vi "Periodic Tasks.vi"(8 "error in (no error)":errorcluster) -> ()   [LabVIEW 2013]
doc: "This VI runs in parallel to other tasks. It can contain as many user-defined periodic loops as you need. These can carry out PID or other sorts of timed response."
uses:
  <vilib>/Rock Robotics/SystemInterfaces/AI/FPGA_AIGyroChannel.ctl
  <vilib>/Rock Robotics/SystemInterfaces/Typedef/FPGA_TypedefAnalogModuleForGyro.ctl
  PnuematicMode.ctl
  TankDriveEnum.ctl
  <vilib>/Rock Robotics/SystemInterfaces/Utilities/FPGA_UtilitiesLED Source.ctl
  <vilib>/Rock Robotics/SystemInterfaces/Utilities/FPGA_UtilitiesLED State.ctl
  Robot Global Data.vi
  <vilib>/Rock Robotics/WPI/Compressor/WPI_CompressorGetSetRefNum.vi
panel:
  out "Angular Rate":dbl
  in  "Analog Module":T1
  in  "Gain (VoltsPerDegree/Second)":dbl=0.007
  in  "Channel":T2
  in  "Reset Zero Position":bool
  out "Angle":dbl(knob) scale=0.0..360.0
  out "error out":errorcluster
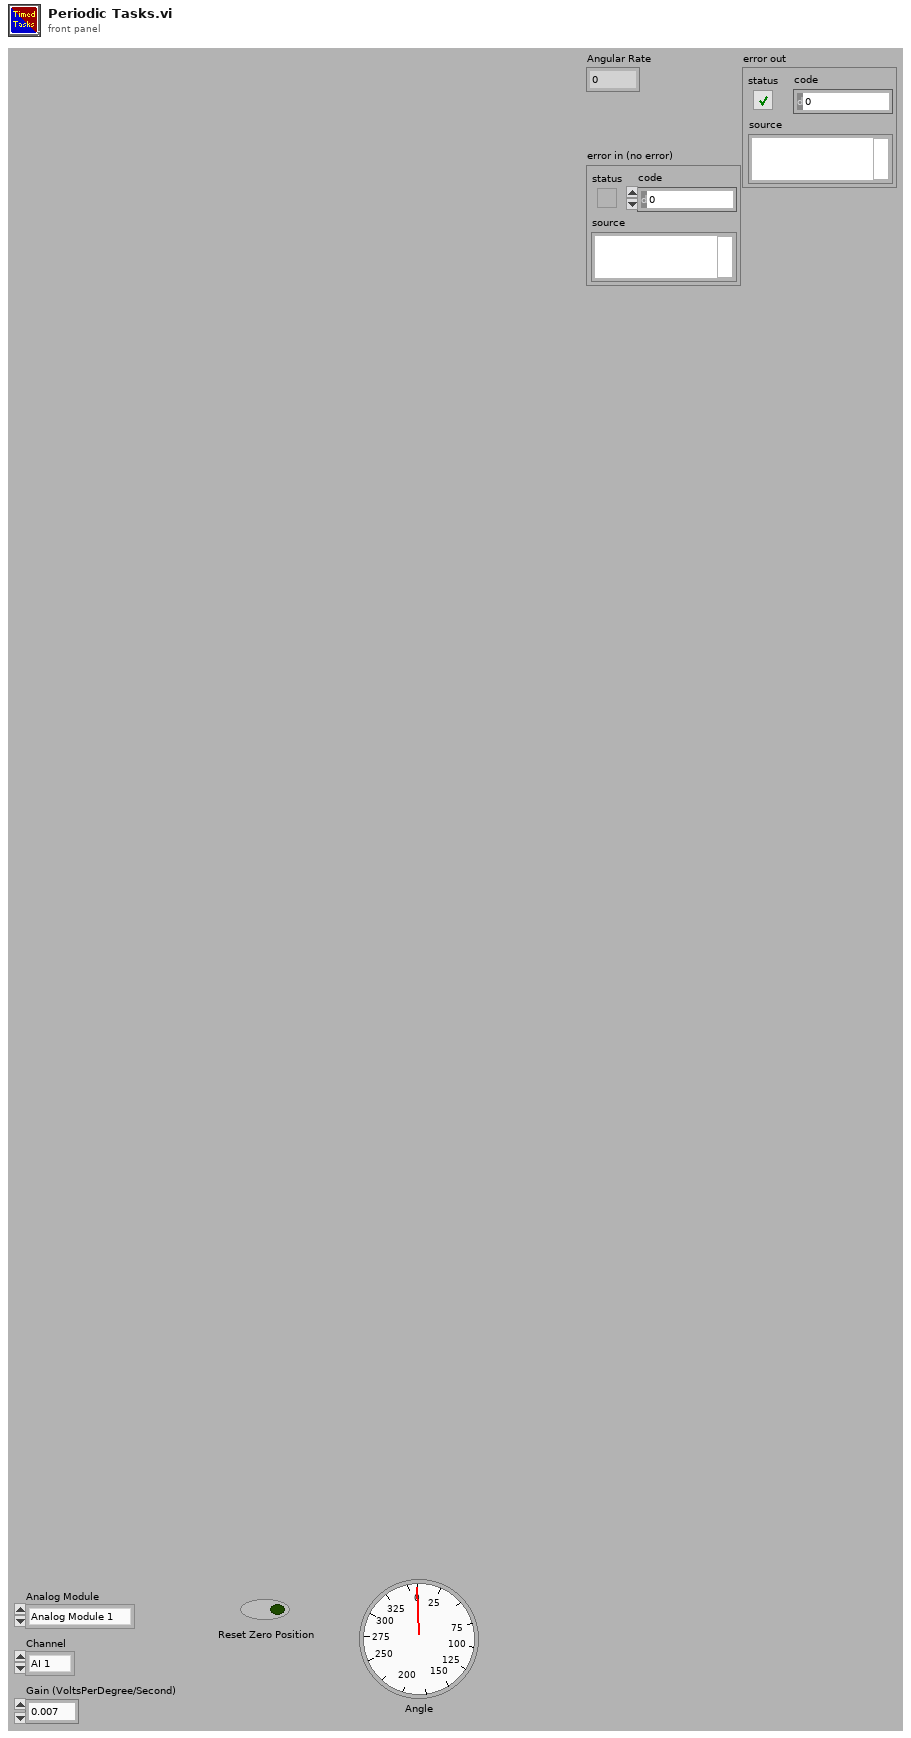
[diagram p1: front panel]
types:
  T1 = typedef "FPGA_TypedefAnalogModuleForGyro.ctl" = enum16{"Analog Module 1"}
  T2 = typedef "FPGA_AIGyroChannel.ctl" = enum8{"AI 1", "AI 2", "Invalid"}
  T3 = typedef "WPI_EncoderDevRef.ctl" = cluster{"DevStatus":errorcluster, "EncoderIndex":T4, "CounterIndex":T5, "DistancePerCount":dbl, "Decoding Type":T6}
  T4 = typedef "FPGA_EncoderIdx.ctl" = enum8{"Enc 0", "Enc 1", "Enc 2", "Enc 3", "Invalid"}
  T5 = typedef "FPGA_CounterCtrSystemIndex.ctl" = enum8{"Ctr 0", "Ctr 1", "Ctr 2", "Ctr 3", "Ctr 4", "Ctr 5", "Ctr 6", "Ctr 7", "Invalid"}
  T6 = typedef "WPI_EncoderType.ctl" = enum16{"1x", "2x", "4x"}
  T7 = typedef "WPI_GyroDevRef.ctl" = cluster{"DevStatus":errorcluster, "Analog Module":T8, "Analog Channel":T9, "Offset":dbl, "Gain (VoltsPerDegree/Second)":dbl}
  T8 = typedef "FPGA_TypedefAnalogModule.ctl" = enum16{"Analog Module 1", "Analog Module 2"}
  T9 = typedef "FPGA_AIChannel.ctl" = enum8{"AI 1", "AI 2", "AI 3", "AI 4", "AI 5", "AI 6", "AI 7", "AI 8", "Invalid"}
  T10 = typedef "WPI_SolenoidDevRef.ctl" = cluster{"DevStatus":errorcluster, "Solenoid Module":T11, "Forward Solenoid Channel":T12, "Reverse Solenoid Channel":T12}
  T11 = typedef "FPGA_TypedefSolenoidModule.ctl" = enum16{"Solenoid Module 1", "Solenoid Module 2"}
  T12 = typedef "WPI_SolenoidChannel.ctl" = enum8{"Solenoid 1", "Solenoid 2", "Solenoid 3", "Solenoid 4", "Solenoid 5", "Solenoid 6", "Solenoid 7", "Solenoid 8", "Invalid"}
  T13 = typedef "WPI_CompressorDevRef.ctl" = cluster{"DevStatus":errorcluster, "DigitalInputDevRef":T14, "RelayDevRef":T17}
  T14 = typedef "WPI_DigitalInputDevRef.ctl" = cluster{"DevStatus":errorcluster, "DIO Channel":T15, "Digital Module":T16}
  T15 = typedef "FPGA_DIOChannel.ctl" = enum8{"DIO 1", "DIO 2", "DIO 3", "DIO 4", "DIO 5", "DIO 6", "DIO 7", "DIO 8", "DIO 9", "DIO 10", "DIO 11", "DIO 12", "DIO 13", "DIO 14", "Invalid"}
  T16 = typedef "FPGA_TypedefDigitalModule.ctl" = enum16{"Digital Module 1", "Digital Module 2"}
  T17 = typedef "WPI_RelayDevRef.ctl" = cluster{"DevStatus":errorcluster, "Relay Channel":T18, "Digital Module":T16, "Relay Direction":T19}
  T18 = typedef "FPGA_DIORelayChannel.ctl" = enum8{"Relay 1", "Relay 2", "Relay 3", "Relay 4", "Relay 5", "Relay 6", "Relay 7", "Relay 8", "Invalid"}
  T19 = typedef "WPI_RelayDirection.ctl" = enum16{"Both directions", "Forward only", "Reverse only"}
  T20 = typedef "TankDriveEnum.ctl" = enum16{"Init", "LinearDrive", "SetValue", "Disable"}
  T21 = typedef "PnuematicMode.ctl" = enum16{"Init", "SetState", "Disable"}
  T22 = typedef "FPGA_UtilitiesLED State.ctl" = enum16{"Off", "On", "Toggle"}
  T23 = typedef "FPGA_UtilitiesLED Source.ctl" = enum16{"User LED", "FPGA LED"}
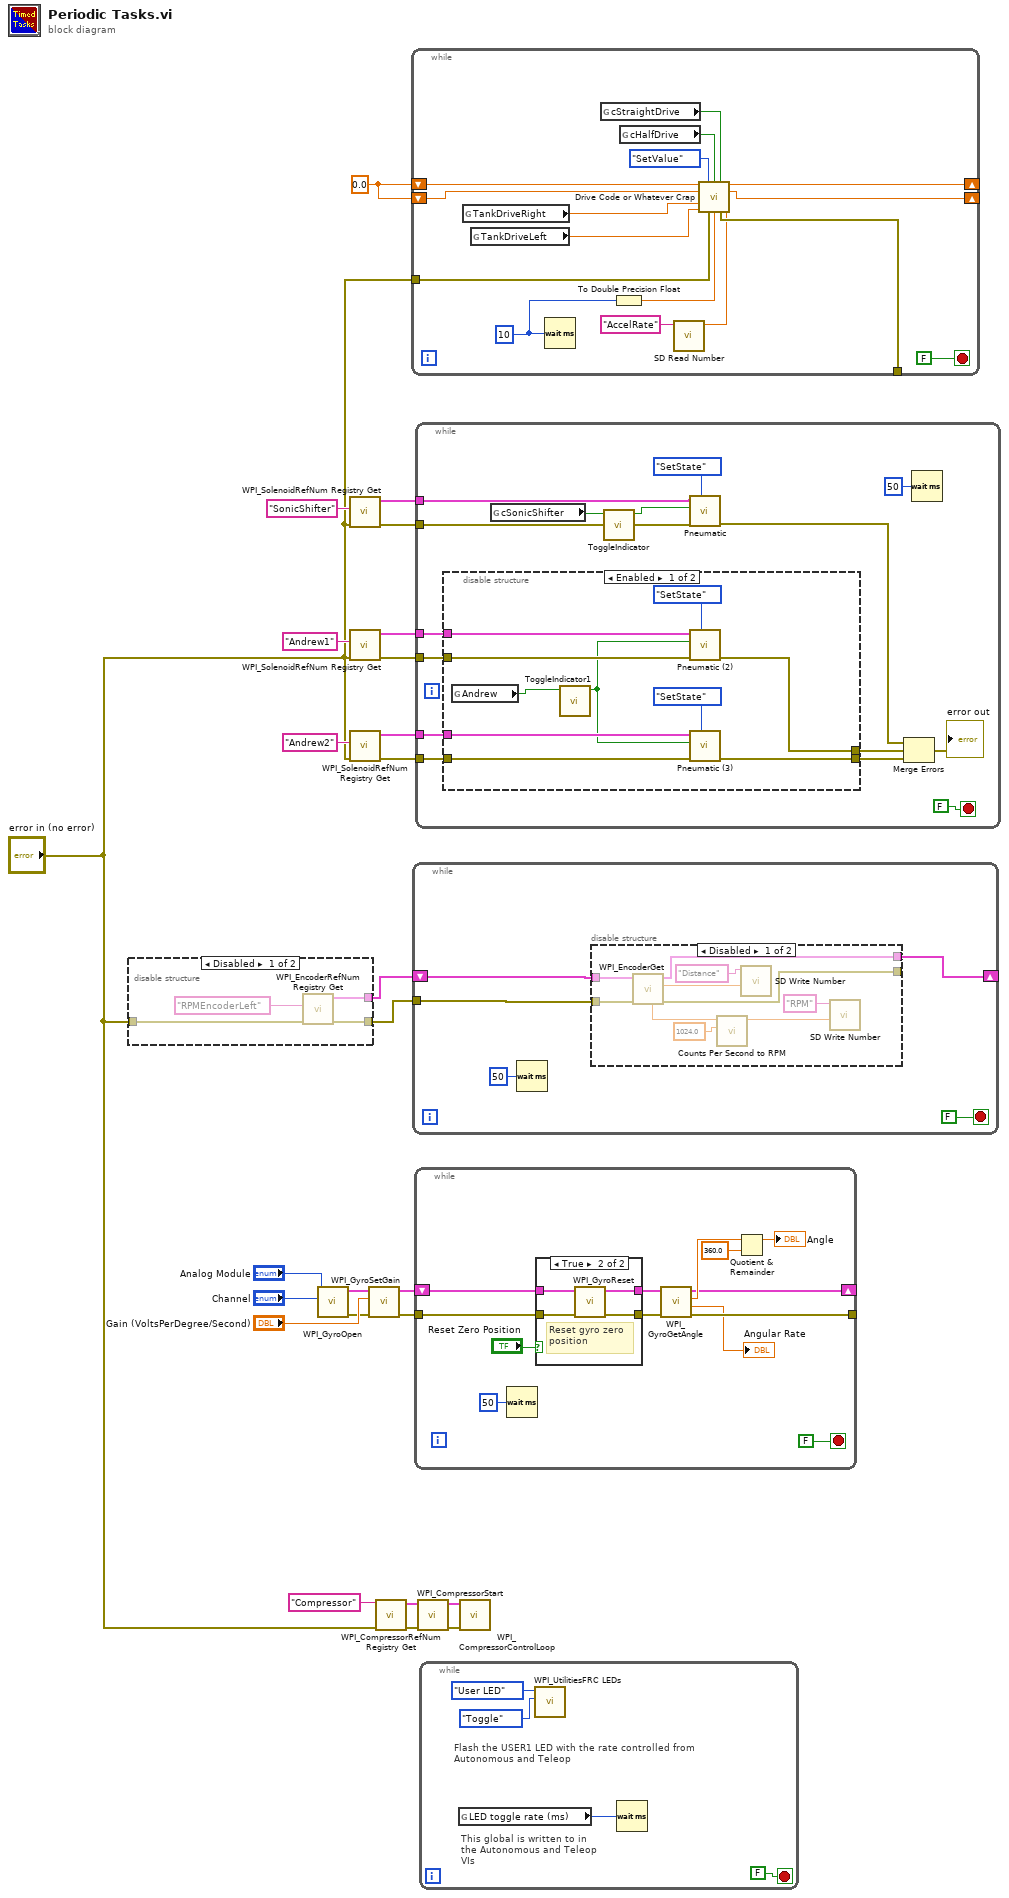
[diagram p0: block diagram]
diagram:
  w11 = 0.0
  n1 = disable-structure shown="Disabled" {
    disable-tunnel: [w28 _] -> w9
    disable-tunnel: [w27 _] -> w8
    disable-tunnel: "error in (no error)" -> [w26 _]
    frame Disabled {
      n2 = call <vilib>:"WPI_EncoderRefNum Registry Get.vi"("error in (no error)"=w26, "refnum name"="RPMEncoderLeft") -> ("error out"=w27:errorcluster, "EncoderDevRef"=w28:T3)  [unwired: 8 in]
    }
    frame Enabled {
    }
  }
  n3 = call <vilib>:"WPI_GyroOpen.vi"("Analog Channel"="Channel", "Analog Module (Module 1)"="Analog Module") -> ("error out"=w2:errorcluster, "GyroDevRef"=w6:T7)  [unwired: 4 in, 4 out]
  n4 = call <vilib>:"WPI_SolenoidRefNum Registry Get.vi"("error in (no error)"="error in (no error)", "refnum name"="SonicShifter") -> ("error out"=w18:errorcluster, "SolenoidDevRef"=w20:T10)  [unwired: 8 in]
  n5 = call <vilib>:"WPI_SolenoidRefNum Registry Get.vi"("error in (no error)"="error in (no error)", "refnum name"="Andrew1") -> ("error out"=w13:errorcluster, "SolenoidDevRef"=w15:T10)  [unwired: 8 in]
  n6 = call <vilib>:"WPI_SolenoidRefNum Registry Get.vi"("error in (no error)"="error in (no error)", "refnum name"="Andrew2") -> ("error out"=w12:errorcluster, "SolenoidDevRef"=w14:T10)  [unwired: 8 in]
  n7 = call <vilib>:"WPI_GyroSetGain.vi"("error in (no error)"=w2, "Gain (VoltsPerDegree/Second)"="Gain (VoltsPerDegree/Second)", "GyroDevRef"=w6) -> ("error out"=w1:errorcluster, "GyroDevRef"=w5:T7)  [unwired: 7 out]
  n8 = call <vilib>:"WPI_CompressorRefNum Registry Get.vi"("error in (no error)"="error in (no error)", "refnum name"="Compressor") -> ("error out"=w22:errorcluster, "CompressorDevRef"=w25:T13)  [unwired: 8 in]
  n9 = while {
    shift-right: [w39] -> _
    shift-left: w11 -> [w40]
    shift-right: [w38] -> _
    shift-left: w11 -> [w41]
    tunnel: "error in (no error)" -> [w37]
    tunnel: [w36] -> _
    stop <- FALSE stop-if-true
    w35 = u32 10 ("milliseconds to wait")
    n10 = global read "Robot Global Data.vi" "TankDriveRight"() -> (w45:dbl)
    n11 = global read "Robot Global Data.vi" "TankDriveLeft"() -> (w44:dbl)
    n12 = Wait (ms)(milliseconds to wait=w35) -> ()  [unwired: 1 out]
    n13 = global read "Robot Global Data.vi" "cStraightDrive"() -> (w42:bool)
    n14 = To Double Precision Float(number=w35) -> (double precision float=w34:dbl)
    n15 = global read "Robot Global Data.vi" "cHalfDrive"() -> (w43:bool)
    n16 = call <vilib>:"SD Read Number.vi"("Name"="AccelRate") -> ("Numeric"=w31:dbl)  [unwired: 8 in, 2 out]
    n17 = call "Drive Code or Whatever Crap.vi"("Right Actual"=w40, "TankDriveEnum"=TankDriveEnum."SetValue" ("Enum"), "HalfDrive"=w43, "StraightDrive"=w42, "LeftActual"=w41, "RightDesired"=w45, "LeftDesired"=w44, "error in (no error)"=w37, "LoopTime"=w34, "AccelRate"=w31) -> ("RightOut"=w39:dbl, "LeftOut"=w38:dbl, "error out"=w36:errorcluster)  [unwired: 3 in]
  }
  n18 = while {
    tunnel: w8 -> [w47]
    shift-right: [w46] -> _
    shift-left: w9 -> [w48]
    stop <- FALSE stop-if-true
    n19 = Wait (ms)(milliseconds to wait=u32 50) -> ()  [unwired: 1 out]
    n20 = disable-structure shown="Disabled" {
      disable-tunnel: w47 -> [w60 _]
      disable-tunnel: w48 -> [w53 _]
      disable-tunnel: [w52 _] -> _
      disable-tunnel: [w51 _] -> w46
      frame Disabled {
        n21 = call <vilib>:"WPI_EncoderGet.vi"("error in (no error)"=w60, "EncoderDevRef"=w53) -> ("error out"=w52:errorcluster, "Distance"=w55:dbl, "EncoderDevRef"=w51:T3, "Rate"=w59:dbl)  [unwired: 4 in, 2 out]
        n22 = call "Counts Per Second to RPM.vi"("Counts/Rev"=1024.0, "Counts/Second"=w59) -> ("RPM"=w57:dbl)  [unwired: 9 in]
        n23 = call <vilib>:"SD Write Number.vi"("Numeric"=w55, "Name"="Distance") -> ()  [unwired: 8 in, 2 out]
        n24 = call <vilib>:"SD Write Number.vi"("Numeric"=w57, "Name"="RPM") -> ()  [unwired: 8 in, 2 out]
      }
      frame Enabled {
      }
    }
  }
  n25 = while {
    shift-right: [w69] -> _
    shift-left: w5 -> [w72]
    tunnel: w1 -> [w65]
    tunnel: [w63] -> _
    stop <- FALSE stop-if-true
    n26 = Wait (ms)(milliseconds to wait=u32 50) -> ()  [unwired: 1 out]
    n27 = case shown="True" "Reset Zero Position" {
      tunnel: w72 -> [w74 w78]
      tunnel: [w74 w77] -> w71
      tunnel: w65 -> [_ w76]
      tunnel: [_ w75] -> w64
      frame False {
      }
      frame True {
        # "Reset gyro zero \nposition"
        n28 = call <vilib>:"WPI_GyroReset.vi"("error in (no error)"=w76, "GyroDevRef"=w78) -> ("error out"=w75:errorcluster, "GyroDevRef"=w77:T7)  [unwired: 8 out]
      }
    }
    n29 = call <vilib>:"WPI_GyroGetAngle.vi"("error in (no error)"=w64, "GyroDevRef"=w71) -> ("error out"=w63:errorcluster, "Angular Rate"=→"Angular Rate":dbl, "Angle"=w70:dbl, "GyroDevRef"=w69:T7)  [unwired: 6 out]
    n30 = Quotient & Remainder(x=w70, y=360.0) -> (x-y*floor(x/y)=→"Angle":dbl)  [unwired: 1 out]
  }
  n31 = while {
    tunnel: w20 -> [w91]
    tunnel: w18 -> [w92]
    tunnel: w15 -> [w87]
    tunnel: w14 -> [w86]
    tunnel: w13 -> [w89]
    tunnel: w12 -> [w85]
    stop <- FALSE stop-if-true
    n32 = disable-structure shown="Enabled" {
      disable-tunnel: w89 -> [w103 _]
      disable-tunnel: [w102 _] -> w88
      disable-tunnel: w87 -> [w101 _]
      disable-tunnel: w86 -> [w99 _]
      disable-tunnel: w85 -> [w98 _]
      disable-tunnel: [w97 _] -> w84
      frame Enabled {
        n33 = global read "Robot Global Data.vi" "Andrew"() -> (w95:bool)
        n34 = call "ToggleIndicator1.vi"("cSonicShifter"=w95) -> ("Actuate?"=w94:bool)  [unwired: 10 in]
        n35 = call "Pneumatic (2).vi"("Mode"=PnuematicMode."SetState", "error in (no error)"=w103, "State"=w94, "SolenoidDevRef"=w101) -> ("error out"=w102:errorcluster)  [unwired: 7 in]
        n36 = call "Pneumatic (3).vi"("Mode"=PnuematicMode."SetState", "error in (no error)"=w98, "State"=w94, "SolenoidDevRef"=w99) -> ("error out"=w97:errorcluster)  [unwired: 7 in]
      }
      frame Disabled {
      }
    }
    n37 = global read "Robot Global Data.vi" "cSonicShifter"() -> (w83:bool)
    n38 = call "ToggleIndicator.vi"("cSonicShifter"=w83) -> ("Actuate?"=w82:bool)  [unwired: 10 in]
    n39 = call "Pneumatic.vi"("Mode"=PnuematicMode."SetState", "error in (no error)"=w92, "State"=w82, "SolenoidDevRef"=w91) -> ("error out"=w79:errorcluster)  [unwired: 7 in]
    n40 = Merge Errors(w79, w88, w84) -> (→"error out":errorcluster)
    n41 = Wait (ms)(milliseconds to wait=u32 50) -> ()  [unwired: 1 out]
  }
  n42 = call <vilib>:"WPI_CompressorStart.vi"("error in (no error)"=w22, "CompressorDevRef"=w25) -> ("error out"=w19:errorcluster, "CompressorDevRef"=w24:T13)  [unwired: 8 in]
  n43 = while {
    stop <- FALSE stop-if-true
    # "This global is written to in the Autonomous and Teleop VIs"
    # "Flash the USER1 LED with the rate controlled from Autonomous and Teleop"
    n44 = global read "Robot Global Data.vi" "LED toggle rate (ms)"() -> (w104:u32)
    n45 = call <vilib>:"WPI_UtilitiesFRC LEDs.vi"("State"=FPGA_UtilitiesLED_State."Toggle", "LED Type"=FPGA_UtilitiesLED_Source."User LED") -> ()  [unwired: 1 in, 9 out]
    n46 = Wait (ms)(milliseconds to wait=w104) -> ()  [unwired: 1 out]
  }
  n47 = call <vilib>:"WPI_CompressorControlLoop.vi"("error in (no error)"=w19, "CompressorDevRef"=w24) -> ()  [unwired: 10 in]
